vi "Publish Joystick Data.vi"(10 "Joystick Refnum":string) -> ()   [LabVIEW 2012]
uses:
  <vilib>/Rock Robotics/WPI/Joystick/WPI_JoystickGetSetRefNum.vi
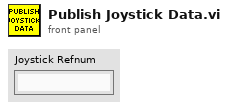
[diagram p1: front panel]
types:
  T1 = typedef "WPI_JoystickDevRef.ctl" = cluster{"Device":T2}
  T2 = typedef "WPI_JoystickDeviceEnum.ctl" = enum16{"USB 1", "USB 2", "USB 3", "USB 4", "Kinect 1", "Kinect 2"}
  T3 = typedef "WPI_JoystickButtonState.ctl" = cluster{"Button 1":bool, "Button 2":bool, "Button 3":bool, "Button 4":bool, "Button 5":bool, "Button 6":bool, "Button 7":bool, "Button 8":bool, "Button 9":bool, "Button 10":bool, "Button 11":bool, "Button 12":bool}
  T4 = cluster{"axis 1 (x)":dbl, "axis 2 (y)":dbl, "axis 3 (throttle)":dbl, "axis 4":dbl, "axis 5":dbl, "axis 6":dbl}
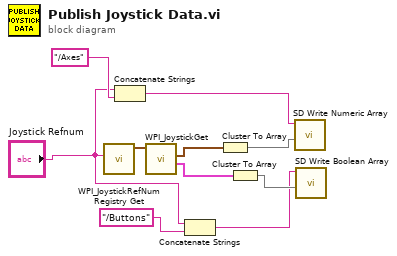
[diagram p0: block diagram]
diagram:
  n1 = call <vilib>:"WPI_JoystickRefNum Registry Get.vi"("refnum name"="Joystick Refnum") -> ("JoystickDevRef"=w10:T1)  [unwired: 1 in, 9 out]
  n2 = Concatenate Strings("Joystick Refnum", "/Axes") -> (w5:string)
  n3 = call <vilib>:"WPI_JoystickGet.vi"("JoystickDevRef"=w10) -> ("Buttons"=w8:T3, "Axes"=w9:T4)  [unwired: 1 in, 4 out]
  n4 = Concatenate Strings("Joystick Refnum", "/Buttons") -> (w1:string)
  n5 = Cluster To Array(cluster=w9) -> (array=w7:dbl[])
  n6 = Cluster To Array(cluster=w8) -> (array=w4:bool[])
  n7 = call <vilib>:"SD Write Numeric Array.vi"("Numeric Array"=w7, "Name"=w5) -> ()  [unwired: 8 in, 2 out]
  n8 = call <vilib>:"SD Write Boolean Array.vi"("Boolean Array"=w4, "Name"=w1) -> ()  [unwired: 8 in, 2 out]
